vi "FRCts20_Backend_Division_GET.vi"(6 "Message Attributes":T4, 8 "error in (no error)":errorcluster, 10 "Data":string, 11 "Engine_Refnums":T1) -> (0 "error out":errorcluster)   [LabVIEW 2014]
doc: "Gets all teams and information under a selected division. Called by the division/team api, and expects a division location."
uses:
  Dependencies/Keyed Array/KeyedArray.ctl
  FRCts20_Backend_EngineRefnums.ctl
  INI_Accessor/FRCts20_Backend_INI Controller.lvclass
  Dependencies/AMC/_SubVIs/TypeDefs/Message Queue.ctl
  Dependencies/AMC/_SubVIs/TypeDefs/Message.ctl
  <vilib>/addons/database/Connection.llb/Conn ObjectReference.ctl
  FRCts20_Backend_FGVOperation.ctl
  FRCts20_Backend_API/FRCts20_Backend_API_Division.ctl
  FRCts20_Backend_API/FRCts20_Backend_API_SW.ctl
  FRCts20_Backend_API/FRCts20_Backend_API_Status.ctl
  FRCts20_Backend_Engine.lvlib
  FRCts20_Backend_API/FRCts20_Backend_API.lvlib
  Dependencies/Keyed Array/Tools_KeyedArray.lvlib
  Dependencies/AMC/AMC.lvlib
  <vilib>/addons/database/NI_Database_API.lvlib
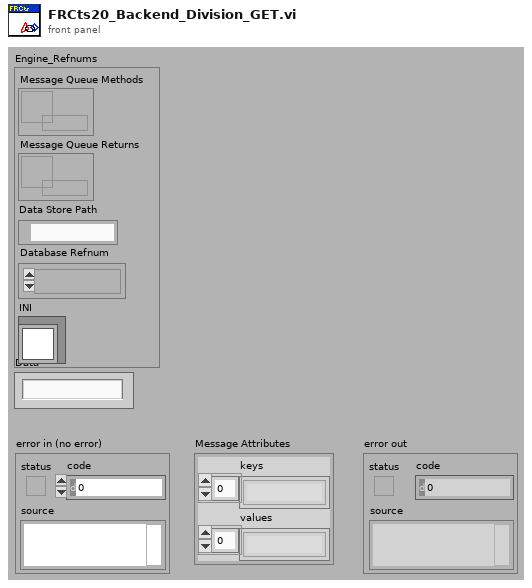
[diagram p1: front panel]
types:
  T1 = typedef "FRCts20_Backend_Engine.lvlib/FRCts20_Backend_EngineRefnums.ctl" = cluster{"Message Queue Methods":T2, "Message Queue Returns":T2, "Data Store Path":path, "Database Refnum":T3, "INI":refnum<class "FRCts20_Backend_INI Controller.lvclass">}
  T2 = typedef "AMC.lvlib/Message Queue.ctl" = refnum<queue>
  T3 = typedef "NI_Database_API.lvlib/Conn ObjectReference.ctl" = refnum<k1>
  T4 = typedef "Tools_KeyedArray.lvlib/KeyedArray.ctl" = cluster{"keys":string[], "values":string[]}
  T5 = typedef "FRCts20_Backend_API.lvlib/FRCts20_Backend_API_Division.ctl" = cluster{"Location":string, "Team":u32[], "APIReturn":string, "RootCmd":enum16{"Issues", "Software", "All"}, "SWType":T6, "Status":T7, "Competition":string}
  T6 = typedef "FRCts20_Backend_API.lvlib/FRCts20_Backend_API_SW.ctl" = string
  T7 = typedef "FRCts20_Backend_API.lvlib/FRCts20_Backend_API_Status.ctl" = enum16{"Open", "In Work", "Closed"}
  T8 = typedef "FRCts20_Backend_Engine.lvlib/FRCts20_Backend_FGVOperation.ctl" = enum16{"Initialize", "EnqueueMessage", "EnqueueDataReturn", "FlushMessage", "FlushDataReturn"}
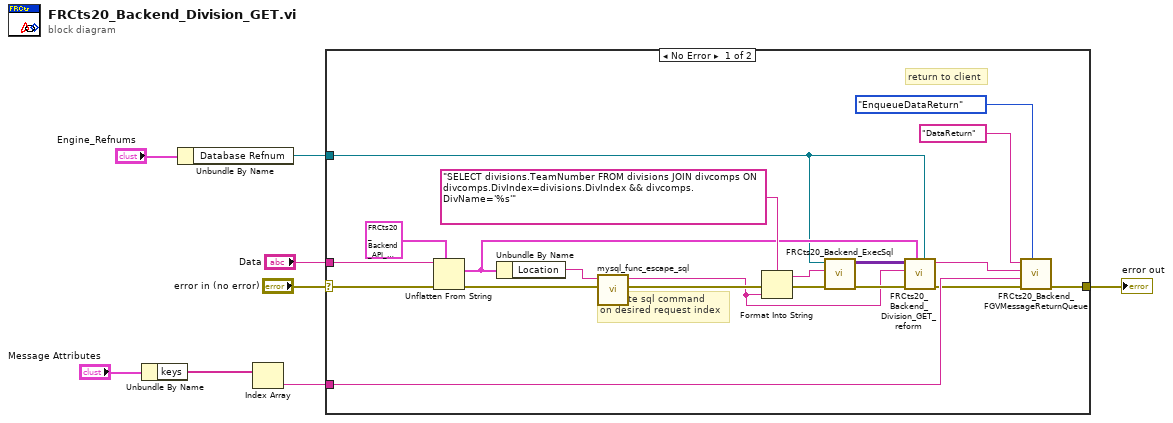
[diagram p0: block diagram]
diagram:
  n1 = Unbundle By Name("Message Attributes") -> ("keys"=w4:string[])
  n2 = Unbundle By Name("Engine_Refnums") -> ("Database Refnum"=w1:T3)
  n3 = Index Array(array=w4) -> (element=w3:string)  [unwired: 1 in]
  n4 = case shown="No Error" "error in (no error)" {
    selector: "error in (no error)" -> [w25 w29]
    tunnel: [w28 w29] -> w7
    tunnel: w1 -> [w10 _]
    tunnel: "Data" -> [w26 _]
    tunnel: w3 -> [w27 _]
    frame No Error {
      # "return to client"
      # "Execute sql command\non desired request index"
      n5 = Unflatten From String(type=T5 {"Location"="", "Team"=[], "APIReturn"="", "RootCmd"=enum."Issues", "SWType"="", "Status"=enum."Open", "Competition"=""} ("Division"), binary string=w26, error in (no error)=w25) -> (value=w11:T5, error out=w17:errorcluster)  [unwired: 2 in, 1 out]
      n6 = Unbundle By Name(w11) -> ("Location"=w18:string)
      n7 = call "mysql_func_escape_sql.vi"("error in (no error)"=w17, "sqlin"=w18) -> ("error out"=w16:errorcluster, "escaped"=w9:string)  [unwired: 8 in]
      n8 = Format Into String(format string="SELECT divisions.TeamNumber FROM divisions JOIN divcomps ON divcomps.DivIndex=divisions.DivIndex && divcomps.DivName='%s'", error in=w16, w9) -> (resulting string=w14:string, error out=w15:errorcluster)  [unwired: 1 in]
      n9 = call "FRCts20_Backend_ExecSql.vi"("error in (no error)"=w15, "format string"=w14, "Refnum in"=w10) -> ("error out"=w12:errorcluster, "recordset data"=w13:variant[][])  [unwired: 6 in, 1 out]
      n10 = call "FRCts20_Backend_Division_GET_reform.vi"("Refnum in"=w10, 7:"Division"=w11, "error in (no error)"=w12, 10:"Division"=w9, "recordset data"=w13) -> ("error out"=w20:errorcluster, "data string"=w21:string)  [unwired: 5 in]
      n11 = call "FRCts20_Backend_FGVMessageReturnQueue.vi"("Operation"=FRCts20_Backend_FGVOperation."EnqueueDataReturn", "error in (no error)"=w20, "Key"=w27, "Message Value"=w21, "Message Name"="DataReturn") -> ("error out"=w28:errorcluster)  [unwired: 5 in, 1 out]
    }
    frame Error {
    }
  }
  "error out" <- w7
